vi "sub vi - analog 1st setup v1.vi"() -> (1 "Graph 1":dynamicdata(graph), 2 "Graph 2":dynamicdata(graph), 3 "Graph 3":dynamicdata(graph), 10 "loop time":dbl format="%.6g", 15 "error out":errorcluster)   [LabVIEW 2013]
panel:
  in  "Tab Control":enum32{"Page 1", "Page 2", "Page 3"}(tab)
  # "RUN THIS VERSION WITH ANALOG INPUT SET TO FALSE TO KICK START EXPRESS VI'S"
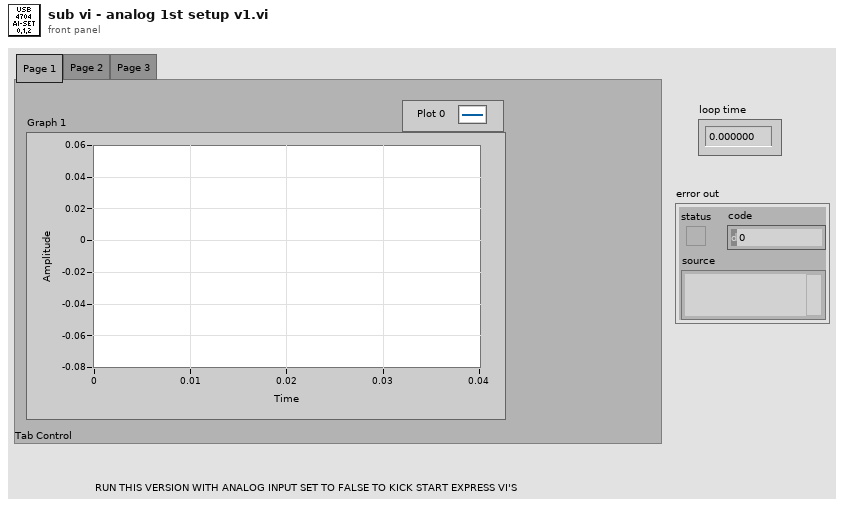
[diagram p1: front panel]
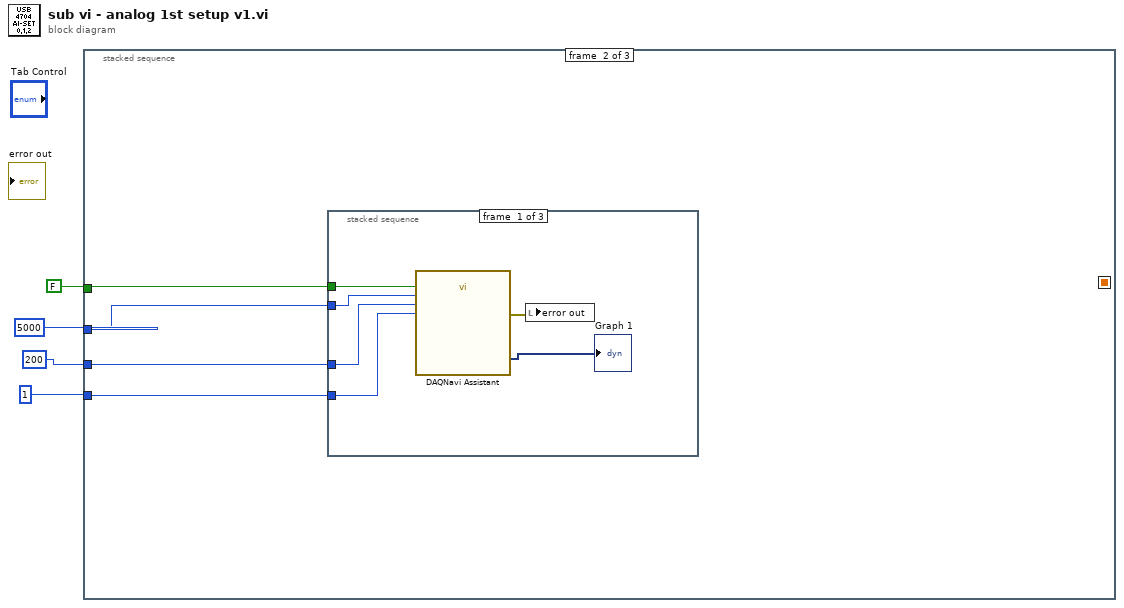
[diagram p0: block diagram]
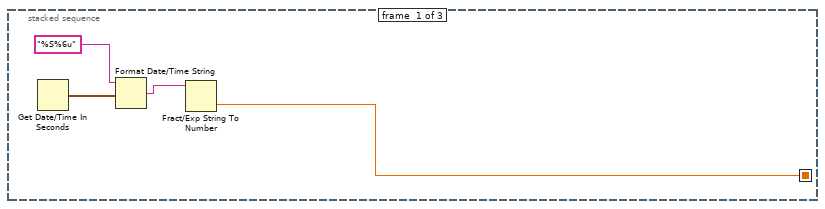
[diagram p2: hidden frame]
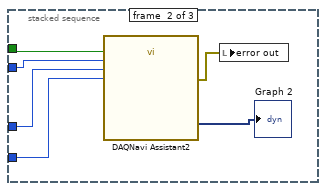
[diagram p3: hidden frame]
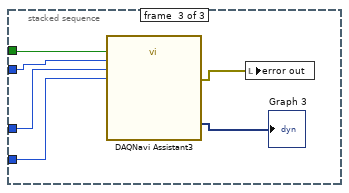
[diagram p4: hidden frame]
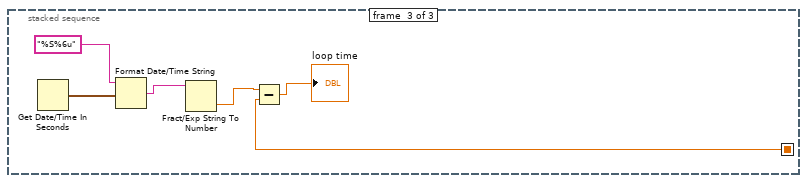
[diagram p5: hidden frame]
diagram:
  n1 = stacked-sequence {
    seq-local: [w5 _ _] -> [_ _ w32]
    tunnel: FALSE -> [_ w12 _]
    tunnel: 1 -> [_ w9 _]
    tunnel: 5000 -> [_ w11 _]
    tunnel: 200 -> [_ w10 _]
    frame #0 {
      n2 = Get Date/Time In Seconds() -> (seconds since 1Jan1904=w7:timestamp)
      n3 = Format Date/Time String(time format string (%c)="%S%6u", seconds (now)=w7) -> (date/time string=w6:string)  [unwired: 1 in]
      n4 = Fract/Exp String To Number(string=w6) -> (number=w5:dbl)  [unwired: 3 in, 1 out]
    }
    frame #1 {
      n5 = stacked-sequence {
        tunnel: w12 -> [w16 w22 w28]
        tunnel: w11 -> [w15 w21 w27]
        tunnel: w10 -> [w14 w20 w26]
        tunnel: w9 -> [w13 w19 w25]
        frame #0 {
          n6 = call "DAQNavi Assistant"("stop(true)"=w16, "conversion rate(Hz)"=w15, "samples"=w14, "time out(10s)"=w13) -> ("error out"=w17:errorcluster, "data out(DDT)"=→"Graph 1":dynamicdata)  [unwired: 22 in]
          n7 = local write "error out"(w17) -> ()
        }
        frame #1 {
          n8 = call "DAQNavi Assistant2"("stop(true)"=w22, "conversion rate(Hz)"=w21, "samples"=w20, "time out(10s)"=w19) -> ("error out"=w24:errorcluster, "data out(DDT)"=→"Graph 2":dynamicdata)  [unwired: 22 in]
          n9 = local write "error out"(w24) -> ()
        }
        frame #2 {
          n10 = call "DAQNavi Assistant3"("stop(true)"=w28, "conversion rate(Hz)"=w27, "samples"=w26, "time out(10s)"=w25) -> ("error out"=w29:errorcluster, "data out(DDT)"=→"Graph 3":dynamicdata)  [unwired: 22 in]
          n11 = local write "error out"(w29) -> ()
        }
      }
    }
    frame #2 {
      n12 = Get Date/Time In Seconds() -> (seconds since 1Jan1904=w35:timestamp)
      n13 = Format Date/Time String(time format string (%c)="%S%6u", seconds (now)=w35) -> (date/time string=w34:string)  [unwired: 1 in]
      n14 = Fract/Exp String To Number(string=w34) -> (number=w33:dbl)  [unwired: 3 in, 1 out]
      n15 = Subtract(x=w33, y=w32) -> (x-y=→"loop time":dbl)
    }
  }
